vi "DemoClass1_GetClassAttributes.vi"(0 "reference in":refnum<class "DemoClass1.lvclass">, 5 "error in (no error)":errorcluster) -> (14 "reference out":refnum<class "DemoClass1.lvclass">, 16 "Class attributes":T1, 17 "Attributes locked?":bool, 19 "error out":errorcluster)   [LabVIEW 2020, in "DemoClass1.lvclass"]
doc: "Returns the class attributes of this class or a sub class. If reference is wired, the class attributes of the class (or sub class) will be returned else the class attributes will default to this class.\n\nIf the data is currently locked for modification, 'Attributes locked?' will return TRUE. If reference is wired, the class attributes of this class (or sub class) will be returned else the class attributes of this class."
uses:
  <vilib>/addons/GOOPUtility/_Demo/GOOPUtil_Demo/DemoClass1_class/DemoClass1.lvclass
  <vilib>/addons/GOOPUtility/_Demo/GOOPUtil_Demo/DemoClass1_class/protected/ClassAttributes.ctl
  <vilib>/addons/_goop3.llb/3GOOPStates.ctl
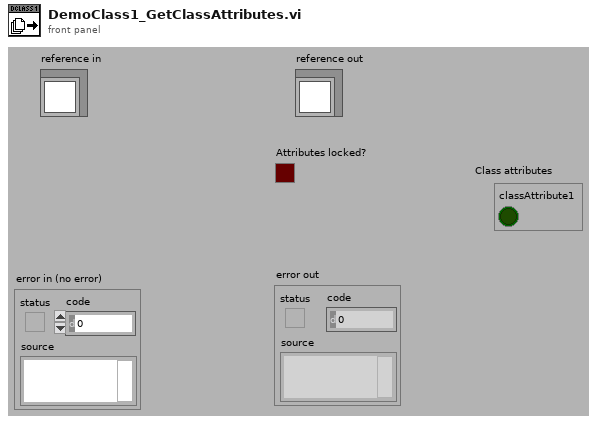
[diagram p1: front panel]
types:
  T1 = typedef "DemoClass1.lvclass/ClassAttributes.ctl" = cluster{"classAttribute1":bool}
  T2 = typedef "3GOOPStates.ctl" = enum16{"Set", "Get", "New", "Delete", "Clear", "Test and get", "Unlock data", "Information", "Look up existing", "New or look up existing", "Test and get shared", "Get shared", "Set shared", "Unlock shared", "Find dynamic method", "Register dynamic method", "Preload dynamic method", "Probe", "Cast to more generic", "Cast to more specific"}
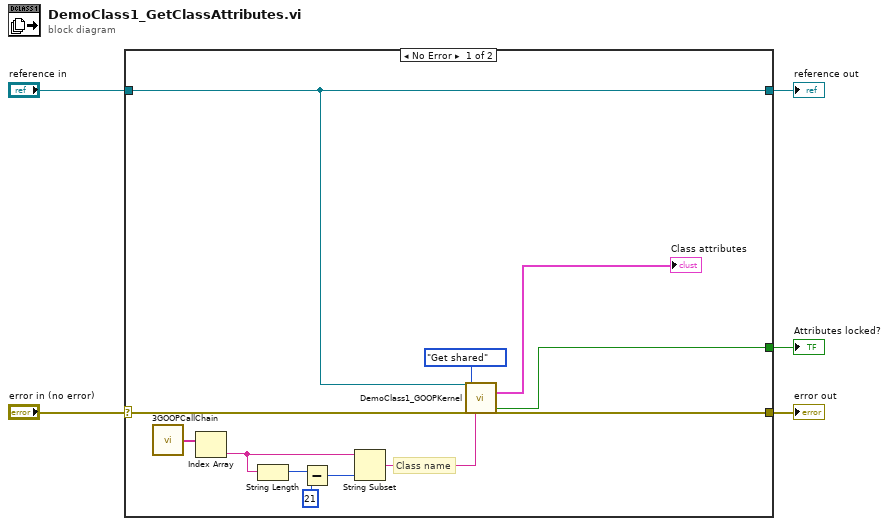
[diagram p0: block diagram]
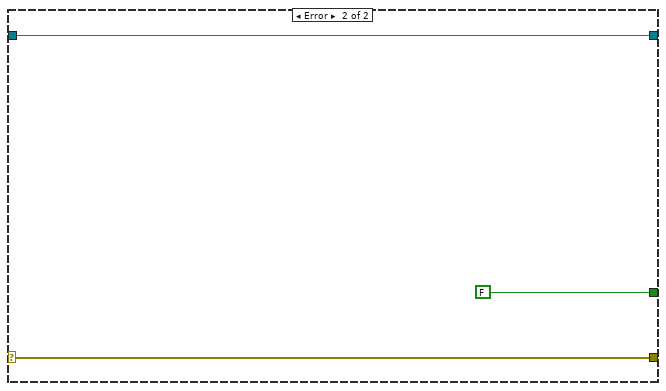
[diagram p2: hidden frame]
diagram:
  n1 = case shown="No Error" "error in (no error)" {
    selector: "error in (no error)" -> [w15 w19]
    tunnel: [w6 w20] -> w5
    tunnel: [w17 w19] -> w4
    tunnel: "reference in" -> [w6 w20]
    tunnel: [w16 FALSE ("Data locked?")] -> w1
    frame No Error {
      # "Class name"
      n2 = call <vilib>:"3GOOPCallChain.vi"() -> ("call chain"=w10:string[])
      n3 = Index Array(array=w10) -> (element=w7:string)  [unwired: 1 in]
      n4 = String Length(string=w7) -> (length=w12:i32)
      n5 = Subtract(x=w12, y=21) -> (x-y=w9:i32)
      n6 = String Subset(string=w7, length (rest)=w9) -> (substring=w8:string)  [unwired: 1 in]
      n7 = call <vilib>:"DemoClass1_GOOPKernel.vi"("Ref in"=w6, "error in (no error)"=w15, "Action"=3GOOPStates."Get shared", "Class name"=w8) -> ("Data shared out"=→"Class attributes":T1, "Data locked?"=w16:bool, "error out"=w17:errorcluster)  [unwired: 13 in, 8 out]
    }
    frame Error {
    }
  }
  "error out" <- w4
  "reference out" <- w5
  "Attributes locked?" <- w1
